vi "Find Pane.vi"(8 "error in":errorcluster, 10 "VI":refnum<vi>) -> (0 "error out":errorcluster, 2 "Pane Ref":refnum<vi>)   [LabVIEW 2020, in "_Rescript.lvlib"]
uses:
  _Rescript.lvlib
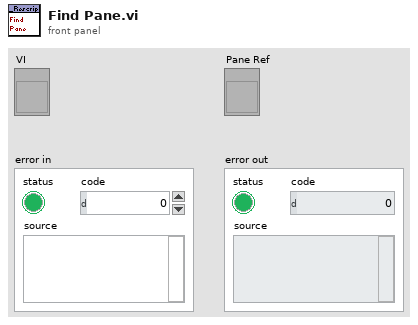
[diagram p1: front panel]
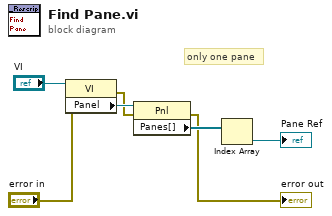
[diagram p0: block diagram]
diagram:
  # "only one pane"
  n1 = property class="VI"(reference="VI", error in="error in") -> (error out=w5:errorcluster, "Panel"=w7:refnum<vi>)  [unwired: 1 out]
  n2 = property class="Pnl"(reference=w7, error in=w5) -> (error out=→"error out":errorcluster, "Panes[]"=w6:refnum<vi>[])  [unwired: 1 out]
  n3 = Index Array(array=w6) -> (element=→"Pane Ref":refnum<vi>)  [unwired: 1 in]
